vi "Determine Warnings - Reusable subVIs.vi"(6 "강풍":dbl, 7 "풍속":dbl, 8 "에러 입력(에러 없음)":errorcluster, 9 "최저 온도":dbl, 10 "최고 온도":dbl, 11 "온도":dbl) -> (0 "에러 출력":errorcluster, 1 "정지":bool, 2 "텍스트":string)   [LabVIEW 2010]
doc: "이것은 LabVIEW Core II에서 사용되는 연습문제 VI입니다. 개선할 필요가 있는 상속된 코드의 예입니다. VI를 기능상의 변경없이 읽기 쉽고 관리하기 쉽도록 만드십시오."
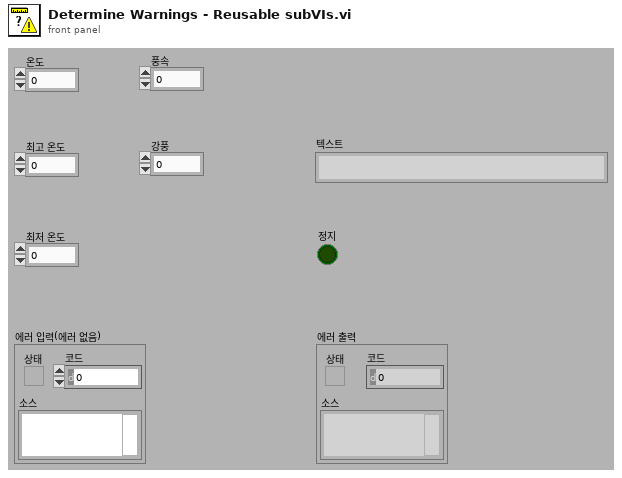
[diagram p1: front panel]
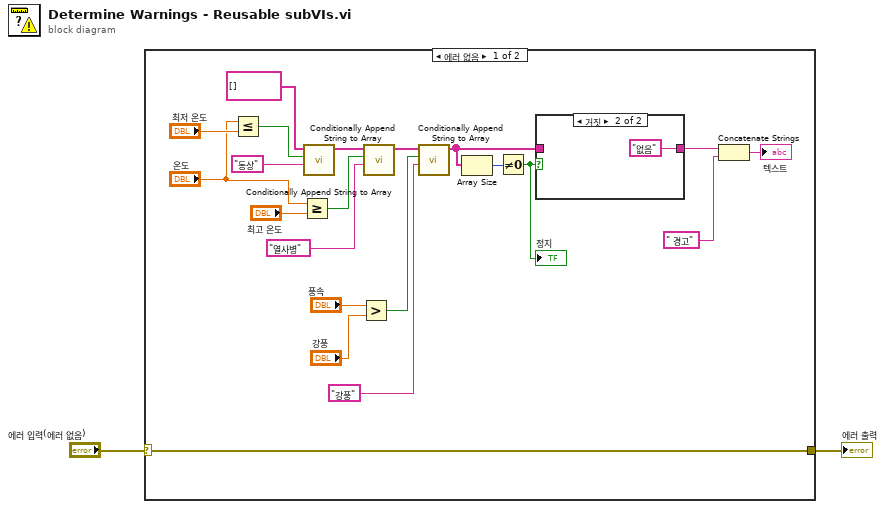
[diagram p0: block diagram]
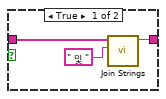
[diagram p2: hidden frame]
diagram:
  n1 = case shown="에러 없음" "에러 입력(에러 없음)" {
    selector: "에러 입력(에러 없음)" -> [w3 w28]
    tunnel: [w3 w28] -> w1
    frame No Error {
      n2 = Less Or Equal?(x="온도", y="최저 온도") -> (x <= y?=w18:bool)
      n3 = Greater Or Equal?(x="온도", y="최고 온도") -> (x >= y?=w13:bool)
      n4 = call "Conditionally Append String to Array.vi"("배열에 추가할 텍스트"="동상", "추가?"=w18, "문자열 배열 입력"=string[] []) -> ("문자열 배열 출력"=w15:string[])  [unwired: 8 out]
      n5 = Greater?(x="풍속", y="강풍") -> (0:w11:bool)
      n6 = call "Conditionally Append String to Array.vi"("배열에 추가할 텍스트"="열사병", "추가?"=w13, "문자열 배열 입력"=w15) -> ("문자열 배열 출력"=w14:string[])  [unwired: 8 out]
      n7 = call "Conditionally Append String to Array.vi"("배열에 추가할 텍스트"="강풍", "추가?"=w11, "문자열 배열 입력"=w14) -> ("문자열 배열 출력"=w9:string[])  [unwired: 8 out]
      n8 = Array Size(array=w9) -> (size(s)=w8:i32)
      n9 = Not Equal To 0?(x=w8) -> (x != 0?=w7:bool)
      "정지" <- w7
      n10 = case shown="거짓" w7 {
        tunnel: [w25 "없음" ("f")] -> w5
        tunnel: w9 -> [w26 _]
        frame True {
          n11 = call "Join Strings.vi"("구분자 (\", \")"=" 및 " ("delimiter (Tab)"), "문자열"=w26) -> ("합쳐진 문자열"=w25:string)  [unwired: 9 out]
        }
        frame False {
        }
      }
      n12 = Concatenate Strings(w5, " 경고" ("string")) -> (→"텍스트":string)
    }
    frame Error {
    }
  }
  "에러 출력" <- w1
